vi "Set Exposure Parameter.vi"(8 "error in (no error)":errorcluster, 10 "Value":i32, 11 "Stream":refnum<data-value>) -> (0 "error out":errorcluster, 1 "Set Value":i32, 3 "Stream (duplicate)":refnum<data-value>)   [LabVIEW 2020, in "g_ar_toolkit.capture.lvlib" / "CameraStream.lvclass"]
uses:
  CameraStream.lvclass
  CameraStream.lvclass/CameraStream.ctl
  Camera Parameters.ctl
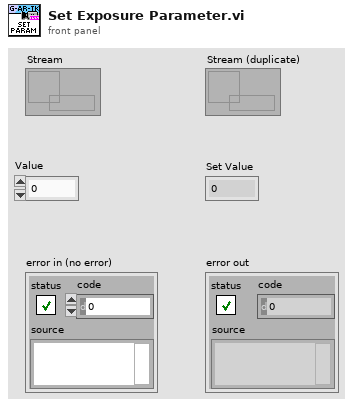
[diagram p1: front panel]
types:
  T1 = typedef "g_ar_toolkit.capture.lvlib/CameraStream.lvclass/Camera Parameters.ctl" = enum8{"EXPOSURE_ABSOLUTE", "FOCUS_ABSOLUTE", "ZOOM_ABSOLUTE", "WHITE_BALANCE_TEMPERATURE", "BRIGHTNESS", "CONTRAST", "SATURATION", "GAMMA", "HUE", "SHARPNESS", "BACKLIGHT_COMPENSATION", "POWER_LINE_FREQUENCY"}
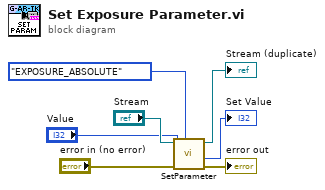
[diagram p0: block diagram]
diagram:
  n1 = call "SetParameter.vi"("Camera Parameter"=Camera_Parameters."EXPOSURE_ABSOLUTE", "error in (no error)"="error in (no error)", "Value"="Value", "Stream"="Stream") -> ("error out"=→"error out":errorcluster, "Set Value"=→"Set Value":i32, "Stream (duplicate)"=→"Stream (duplicate)":refnum<data-value>)  [unwired: 5 in]
